vi "console UI.vi"(10 "to client":refnum<queue>, 11 "from client":refnum<queue>) -> ()   [LabVIEW 2013, in "Websocket console plugin.lvclass"]
uses:
  Websocket console plugin.lvclass
panel:
  in  "stopnmeric":dbl
  in  "send":bool
  in  "out":string
  out "in":string
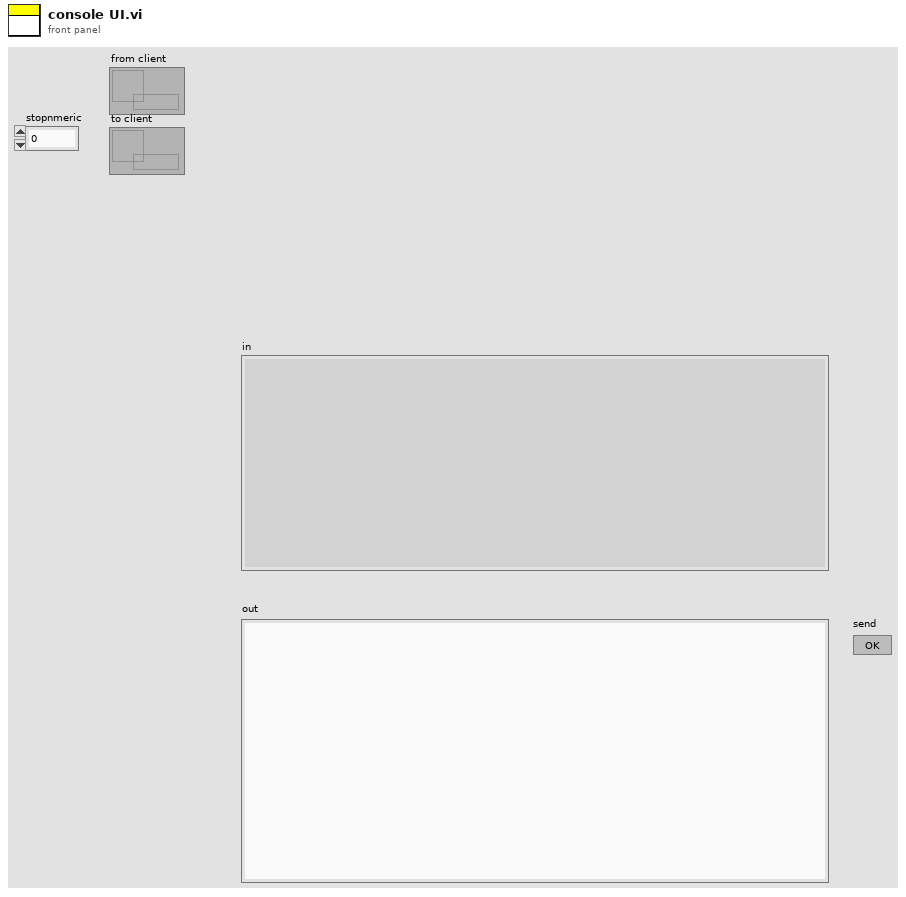
[diagram p1: front panel]
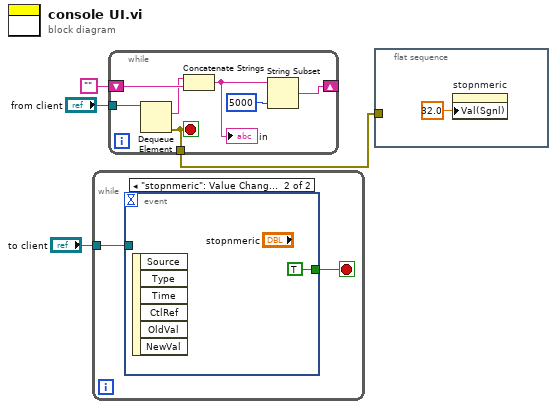
[diagram p0: block diagram]
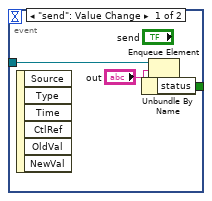
[diagram p2: hidden frame]
diagram:
  n1 = while {
    tunnel: "to client" -> [w6]
    stop <- w5 stop-if-true
    n2 = event shown="[1] \"stopnmeric\": Value Change" {
      selector: _ -> [_ _]
      dyn-events: _ -> [_ _]
      timeout: _ -> [_ _]
      tunnel: w6 -> [w10 _]
      tunnel: [w7 TRUE ("status")] -> w5
      event "send": Value Change {
        n3 = event-data() -> ()  [unwired: 1 in, 6 out]
        n4 = Enqueue Element(queue=w10, element="out") -> (error out=w9:errorcluster)  [unwired: 2 in, 2 out]
        n5 = Unbundle By Name(w9) -> ("status"=w7:bool)
      }
      event "stopnmeric": Value Change {
        n6 = event-data() -> ()  [unwired: 1 in, 6 out]
      }
    }
  }
  n7 = while {
    tunnel: "from client" -> [w18]
    shift-right: [w14] -> _
    shift-left: "" -> [w17]
    tunnel: [w12] -> w1
    stop <- w12 stop-if-true
    n8 = Dequeue Element(queue=w18) -> (element=w16:string, error out=w12:errorcluster)  [unwired: 2 in, 2 out]
    n9 = Concatenate Strings(w16, w17) -> (w15:string)
    "in" <- w15
    n10 = String Subset(string=w15, length (rest)=5000 ("length (rest)")) -> (substring=w14:string)  [unwired: 1 in]
  }
  n11 = flat-sequence {
    tunnel: w1 -> [_]
    frame #0 {
      n12 = property on="stopnmeric" class="DigNum (strict)"("Val(Sgnl)"=32.0 ("Value (Signaling)")) -> ()  [unwired: 2 in, 2 out]
    }
  }
